vi "init.vi"(8 "error in (no error)":errorcluster, 10 "Inputs to Periodic Wave":T1={"Frequency"=10.0, "Amplitude"=1.0, "Phase"=0.0, " Time"=0.0}, 11 "SawtoothWave in":refnum<class "SawtoothWave.lvclass">) -> (0 "error out":errorcluster, 3 "SawtoothWave out":refnum<class "SawtoothWave.lvclass">)   [LabVIEW 2015, in "SawtoothWave.lvclass"]
uses:
  SawtoothWave.lvclass
  Typedefs/PeriodicWaveInputs.ctl
  SawtoothWave.lvclass/SawtoothWave.ctl
  Typedefs/FAMTTypedefs.lvlib
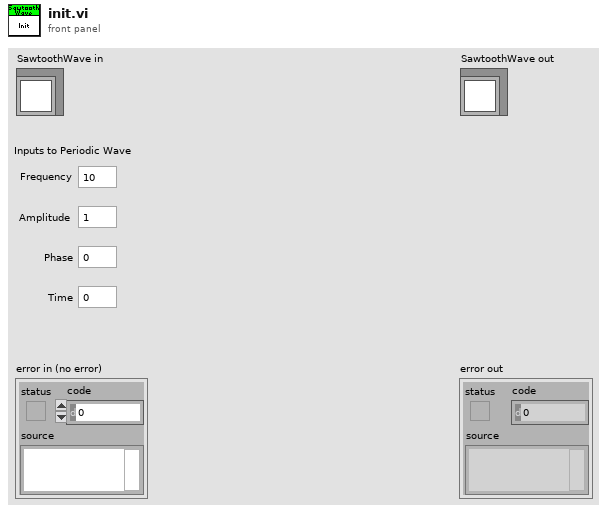
[diagram p1: front panel]
types:
  T1 = typedef "FAMTTypedefs.lvlib/PeriodicWaveInputs.ctl" = cluster{"Frequency":dbl, "Amplitude":dbl, "Phase":dbl, " Time":dbl}
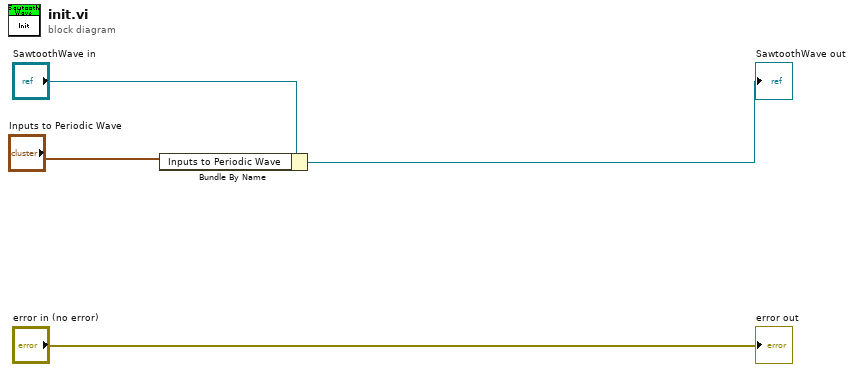
[diagram p0: block diagram]
diagram:
  n1 = Bundle By Name(cluster="SawtoothWave in", "Inputs to Periodic Wave"="Inputs to Periodic Wave") -> (→"SawtoothWave out":refnum<class "SawtoothWave.lvclass">)
  "error out" <- "error in (no error)"
